vi "EXCEL FILE.vi"() -> ()   [LabVIEW 2017]
uses:
  <instrlib>/Agilent 3446X Series/Public/Data/Read (Single Point).vi
  <instrlib>/Agilent 3446X Series/Agilent 3446X Series.lvlib
panel:
  out "Waveform Chart":dbl(graph)
  in  "VISA resource name":refnum<visa-resource-name>
  in  "Auto Range (T: Enable)":bool=TRUE
  in  "Measurement Function (10: Voltage DC)":i32(ring)=10 items=["Continuity", "Current AC", "Current DC", "Diode", "Frequency", "Resistance 4-wire", "Period", "Resistance 2-wire", "Temperature", "Voltage AC", "Voltage DC", "Voltage DC Ratio"]
  out "Measurement":dbl
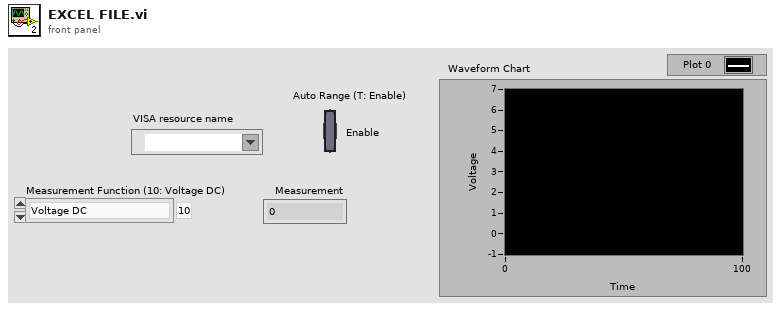
[diagram p1: front panel]
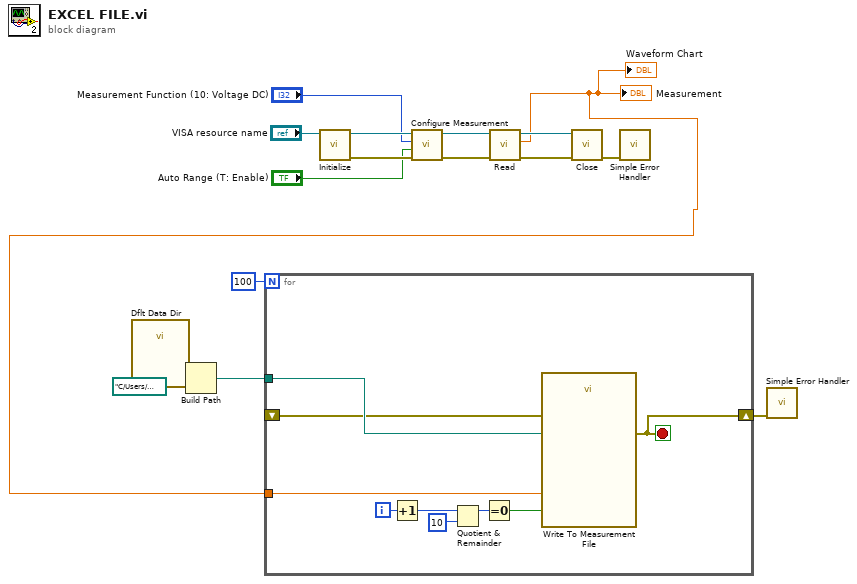
[diagram p0: block diagram]
diagram:
  n1 = call <vilib>:"Dflt Data Dir.vi"() -> ("App:Default Data Directory"=w1:path)  [unwired: 1 in, 3 out]
  n2 = Build Path(base path=w1, name or relative path=path "C:/Users/admin/Documents/LabVIEW Data/test.xlsx" ("default name")) -> (appended path=w3:path)
  n3 = call <instrlib>:"Initialize.vi"("VISA resource name"="VISA resource name") -> ("error out"=w14:errorcluster, "VISA resource name out"=w15:refnum<visa-resource-name>)  [unwired: 4 in, 5 out]
  n4 = call <instrlib>:"Configure Measurement.vi"("error in (no error)"=w14, "Auto Range (T: Enable)"="Auto Range (T: Enable)", "Measurement Function (10: Voltage DC)"="Measurement Function (10: Voltage DC)", "VISA resource name"=w15) -> ("error out"=w10:errorcluster, "VISA resource name out"=w11:refnum<visa-resource-name>)  [unwired: 2 in, 4 out]
  n5 = call-poly <instrlib>:"Read.vi"("error in (no error)"=w10, "VISA resource name"=w11) -> ("error out"=w13:errorcluster, "Measurement"=w2:dbl, "VISA resource name out"=w12:refnum<visa-resource-name>)  [unwired: 7 out]
  "Measurement" <- w2
  "Waveform Chart" <- w2
  n6 = for {
    N: 100 -> [_]
    tunnel: w2 -> [w25]
    shift-right: [w18] -> w6
    shift-left: _ -> [w23]
    tunnel: w3 -> [w24]
    i -> [w22]
    stop <- w18 stop-if-true
    n7 = Increment(x=w22) -> (x+1=w19:i32)
    n8 = Quotient & Remainder(x=w19, y=10) -> (x-y*floor(x/y)=w21:i32)  [unwired: 1 out]
    n9 = Equal To 0?(x=w21) -> (x = 0?=w17:bool)
    n10 = call "Write To Measurement File"("Signals"=w25, "Flush? (T)"=w17, "error in (no error)"=w23, "Filename"=w24) -> ("error out"=w18:errorcluster)  [unwired: 13 in, 2 out]
  }
  n11 = call <instrlib>:"Close.vi"("error in (no error)"=w13, "VISA resource name"=w12) -> ("error out"=w16:errorcluster)  [unwired: 9 out]
  n12 = call <vilib>:"Simple Error Handler.vi"("error in (no error)"=w16) -> ()  [unwired: 1 in, 8 out]
  n13 = call <vilib>:"Simple Error Handler.vi"("error in (no error)"=w6) -> ()  [unwired: 4 in, 5 out]
